vi "Get All Control Refs.vi"(0 "VI Name":string, 1 "vi reference":refnum<vi>, 2 "Type":enum16{"Both", "Controls", "Indicators"}(ring), 3 "Machine Name":string, 4 "Target LV Version #":T1) -> (5 "VI Refnum":refnum<vi>, 6 "All Controls":refnum<vi>[](array[refnum]), 8 "error out":errorcluster)   [LabVIEW 2020]
uses:
  Sub Controls/LV Versions Enum.ctl
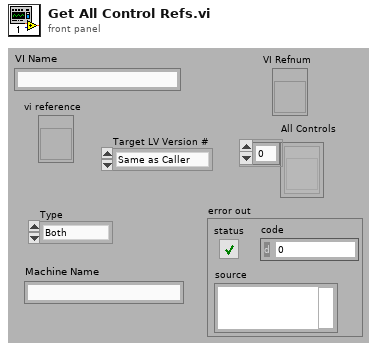
[diagram p1: front panel]
types:
  T1 = typedef "LV Versions Enum.ctl" = enum16{"Same as Caller", "8.0", "8.20", "8.5", "8.6", "9.0", "10.0", "11.0", "12.0", "13.0", "14.0", "15.0", "16.0", "17.0", "18.0", "19.0", "20.0"}
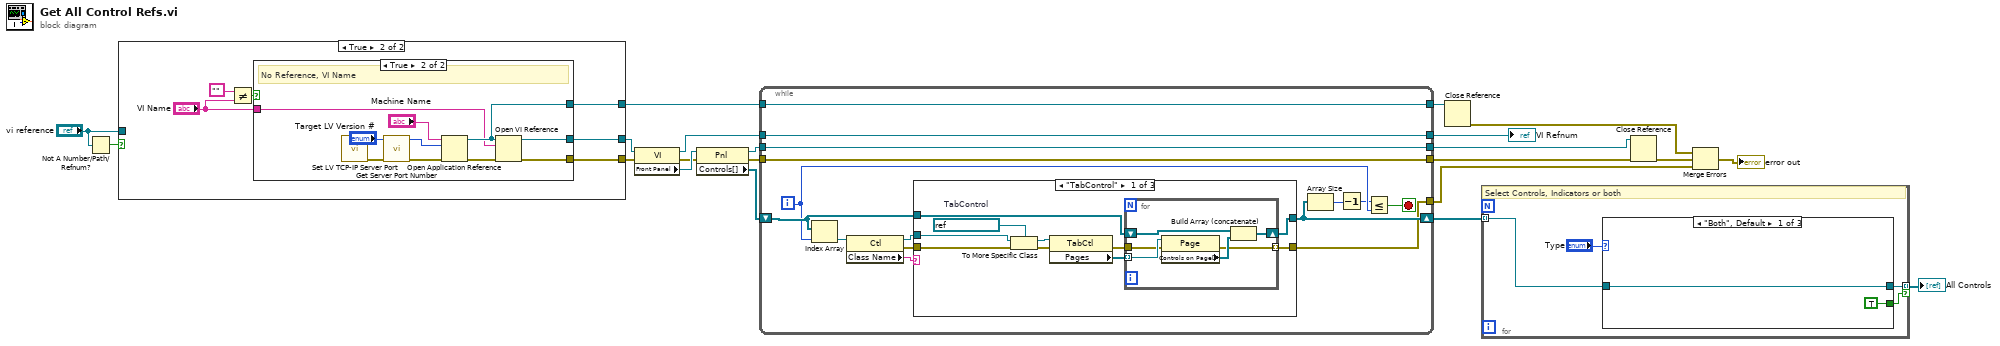
[diagram p0: block diagram]
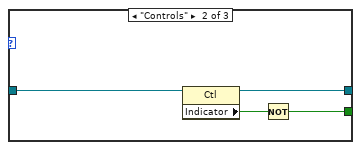
[diagram p2: hidden frame]
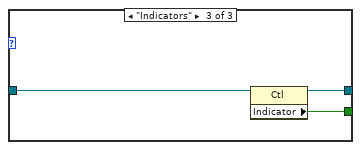
[diagram p3: hidden frame]
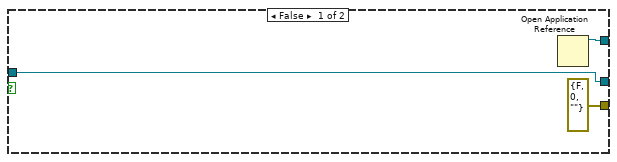
[diagram p4: hidden frame]
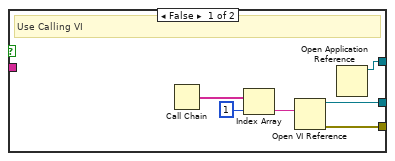
[diagram p5: hidden frame]
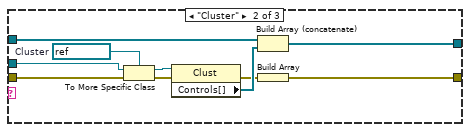
[diagram p6: hidden frame]
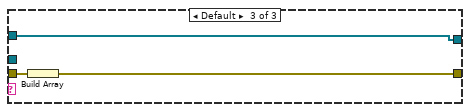
[diagram p7: hidden frame]
diagram:
  n1 = Not A Number/Path/Refnum?(number/path/refnum="vi reference") -> (NaN/Path/Refnum?=w5:bool)
  n2 = case shown="True" w5 {
    tunnel: [w24 w30] -> w21
    tunnel: [errorcluster {"status"=FALSE, "code"=0, "source"=""} ("error out") w29] -> w19
    tunnel: [w22 w28] -> w8
    tunnel: "vi reference" -> [w24 _]
    frame False {
      n3 = Open Application Reference() -> (3:w22:refnum<vi>)  [unwired: 4 in, 1 out]
    }
    frame True {
      n4 = Not Equal?(x="", y="VI Name") -> (x != y?=w25:bool)
      n5 = case shown="True" w25 {
        tunnel: [w35 w46] -> w30
        tunnel: [w34 w45] -> w29
        tunnel: [w36 w43] -> w28
        tunnel: "VI Name" -> [_ w42]
        frame False {
          # "Use Calling VI"
          n6 = Call Chain() -> (call chain=w32:string[])
          n7 = Index Array(array=w32, index=1) -> (element=w31:string)
          n8 = Open VI Reference(vi path=w31) -> (vi reference=w35:refnum<vi>, error out=w34:errorcluster)  [unwired: 5 in]
          n9 = Open Application Reference() -> (3:w36:refnum<vi>)  [unwired: 4 in, 1 out]
        }
        frame True {
          # "No Reference, VI Name"
          n10 = call "Set LV TCP-IP Server Port.vi"() -> ("error out"=w38:errorcluster)  [unwired: 11 in]
          n11 = call "Get Server Port Number.vi"("error in (no error)"=w38, "Target LV Version #"="Target LV Version #") -> ("error out"=w40:errorcluster, "Server Port"=w41:u16)  [unwired: 7 in, 1 out]
          n12 = Open Application Reference(8:w40, 10:w41, 11:"Machine Name") -> (0:w39:errorcluster, 3:w43:refnum<vi>)  [unwired: 1 in]
          n13 = Open VI Reference(application reference (local)=w43, vi path=w42, error in (no error)=w39) -> (vi reference=w46:refnum<vi>, error out=w45:errorcluster)  [unwired: 3 in]
        }
      }
    }
  }
  n14 = property class="VI"(reference=w21, error in=w19) -> (reference out=w9:refnum<vi>, error out=w14:errorcluster, "Front Panel"=w20:refnum<vi>)
  n15 = property class="Pnl"(reference=w20, error in=w14) -> (reference out=w12:refnum<vi>, error out=w10:errorcluster, "Controls[]"=w18:refnum<vi>[])
  n16 = while {
    shift-right: [w60] -> w2
    shift-left: w18 -> [w61]
    tunnel: [w51] -> w16
    tunnel: [w50] -> w13
    tunnel: w12 -> [w50]
    tunnel: w10 -> [w49]
    tunnel: [w49] -> w11
    tunnel: w9 -> [w48]
    tunnel: [w48] -> w6
    tunnel: [w47] -> w7
    tunnel: w8 -> [w47]
    i -> [w58]
    stop <- w57 stop-if-true
    n17 = Index Array(array=w61, index=w58) -> (element=w55:refnum<vi>)
    n18 = property class="Ctl"(reference=w55) -> (reference out=w53:refnum<vi>, error out=w52:errorcluster, "Class Name"=w54:string)  [unwired: 1 in]
    n19 = case shown="\"TabControl\"" w54 {
      tunnel: w61 -> [w70 w87 w90]
      tunnel: [w69 w86 w90] -> w60
      tunnel: w53 -> [w68 w85 _]
      tunnel: w52 -> [w67 w84 w89]
      tunnel: [w62 w78 w88] -> w51
      frame "TabControl" {
        w64 = refnum<vi> refnum  # TabControl
        n20 = To More Specific Class(target class=w64, reference=w68, error in=w67) -> (specific class reference=w65:refnum<vi>, error out=w66:errorcluster)
        n21 = property class="TabCtl"(reference=w65, error in=w66) -> (error out=w63:errorcluster, "Pages"=w71:refnum<vi>[])  [unwired: 1 out]
        n22 = for {
          tunnel: w71 -> [w77] mode=indexing
          shift-right: [w76] -> w69
          shift-left: w70 -> [w75]
          tunnel: w63 -> [w73]
          tunnel: [w72] -> w62 mode=indexing
          n23 = property class="Page"(reference=w77, error in=w73) -> (error out=w72:errorcluster, "Controls on Page[]"=w74:refnum<vi>[])  [unwired: 1 out]
          n24 = Build Array (concatenate)(w75, w74) -> (w76:refnum<vi>[])
        }
      }
      frame "Cluster" {
        w81 = refnum<vi> refnum  # Cluster
        n25 = To More Specific Class(target class=w81, reference=w85, error in=w84) -> (specific class reference=w82:refnum<vi>, error out=w83:errorcluster)
        n26 = property class="Clust"(reference=w82, error in=w83) -> (error out=w79:errorcluster, "Controls[]"=w80:refnum<vi>[])  [unwired: 1 out]
        n27 = Build Array (concatenate)(w87, w80) -> (w86:refnum<vi>[])
        n28 = Build Array(w79) -> (w78:errorcluster[])
      }
      frame Default {
        n29 = Build Array(w89) -> (w88:errorcluster[])
      }
    }
    n30 = Array Size(array=w60) -> (size(s)=w59:i32)
    n31 = Decrement(x=w59) -> (x-1=w56:i32)
    n32 = Less Or Equal?(x=w56, y=w58) -> (x <= y?=w57:bool)
  }
  "VI Refnum" <- w6
  n33 = Close Reference(reference=w7) -> (error out=w1:errorcluster)  [unwired: 1 in]
  n34 = for {
    tunnel: w2 -> [w94] mode=indexing
    tunnel: [w93] -> w3 mode=indexing if=w92
    # "Select Controls, Indicators or both"
    n35 = case shown="\"Both\", Default" "Type" {
      tunnel: w94 -> [w96 w100 w103]
      tunnel: [w96 w99 w102] -> w93
      tunnel: [TRUE ("Indicator") w97 w101] -> w92
      frame "Both", Default {
      }
      frame "Controls" {
        n36 = property class="Ctl"(reference=w100) -> (reference out=w99:refnum<vi>, "Indicator"=w98:bool)  [unwired: 1 in, 1 out]
        n37 = Not(x=w98) -> (.not. x?=w97:bool)
      }
      frame "Indicators" {
        n38 = property class="Ctl"(reference=w103) -> (reference out=w102:refnum<vi>, "Indicator"=w101:bool)  [unwired: 1 in, 1 out]
      }
    }
  }
  "All Controls" <- w3
  n39 = Close Reference(reference=w13, error in (no error)=w11) -> (error out=w15:errorcluster)
  n40 = Merge Errors(w1, w15, w16) -> (→"error out":errorcluster)
